vi "FormVarValuesArray.vi"(2 "varables bytes":i32[](array[numeric]), 3 "varables ports":i32[](array[numeric]), 4 "Ports":u8[](array[numeric])) -> (1 "Values Array":string[](array[string]))   [LabVIEW 2010]
panel:
  out "Boolean array":bool[](array[boolean])
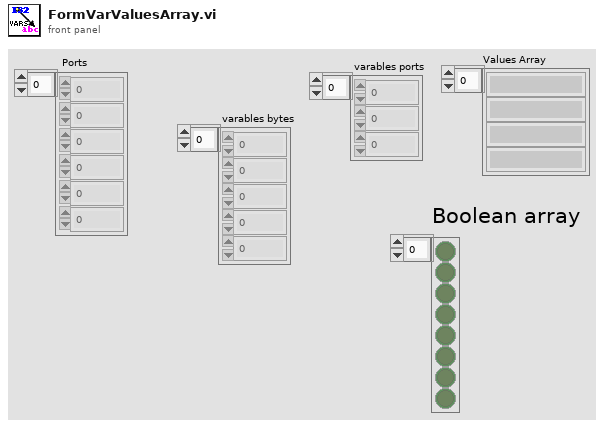
[diagram p1: front panel]
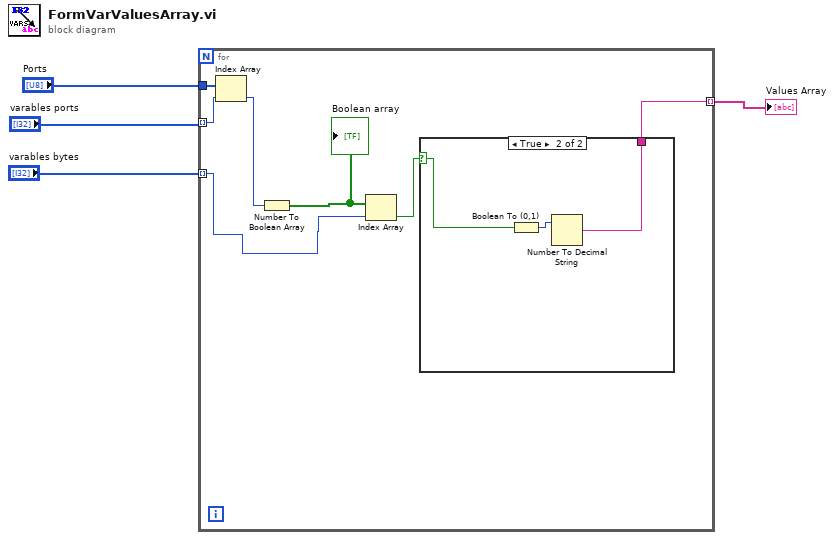
[diagram p0: block diagram]
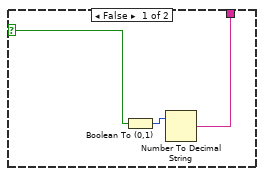
[diagram p2: hidden frame]
diagram:
  n1 = for {
    tunnel: "varables ports" -> [w10] mode=indexing
    tunnel: "Ports" -> [w11]
    tunnel: "varables bytes" -> [w5] mode=indexing
    tunnel: [w9] -> w1 mode=indexing
    n2 = Index Array(array=w11, index=w10) -> (element=w6:u8)
    n3 = Number To Boolean Array(number=w6) -> (Boolean array=w8:bool[])
    "Boolean array" <- w8
    n4 = Index Array(array=w8, index=w5) -> (element=w7:bool)
    n5 = case shown="True" w7 {
      selector: w7 -> [w12 w15]
      tunnel: [w13 w16] -> w9
      frame False {
        n6 = Boolean To (0,1)(Boolean=w12) -> (0, 1=w14:i16)
        n7 = Number To Decimal String(number=w14) -> (decimal integer string=w13:string)  [unwired: 1 in]
      }
      frame True {
        n8 = Boolean To (0,1)(Boolean=w15) -> (0, 1=w17:i16)
        n9 = Number To Decimal String(number=w17) -> (decimal integer string=w16:string)  [unwired: 1 in]
      }
    }
  }
  "Values Array" <- w1
